vi "edit_recepie_1.vi"() -> ()   [LabVIEW 2009]
panel:
  in  "Delete":bool caption="OK2"
  in  "OK":bool caption="OK2"
  in  "Cancel":bool
  in  "path":path=path "D:/System Files/Recipe"
  out "Recipe_path":string
  in  "Recipe":i32(listbox)
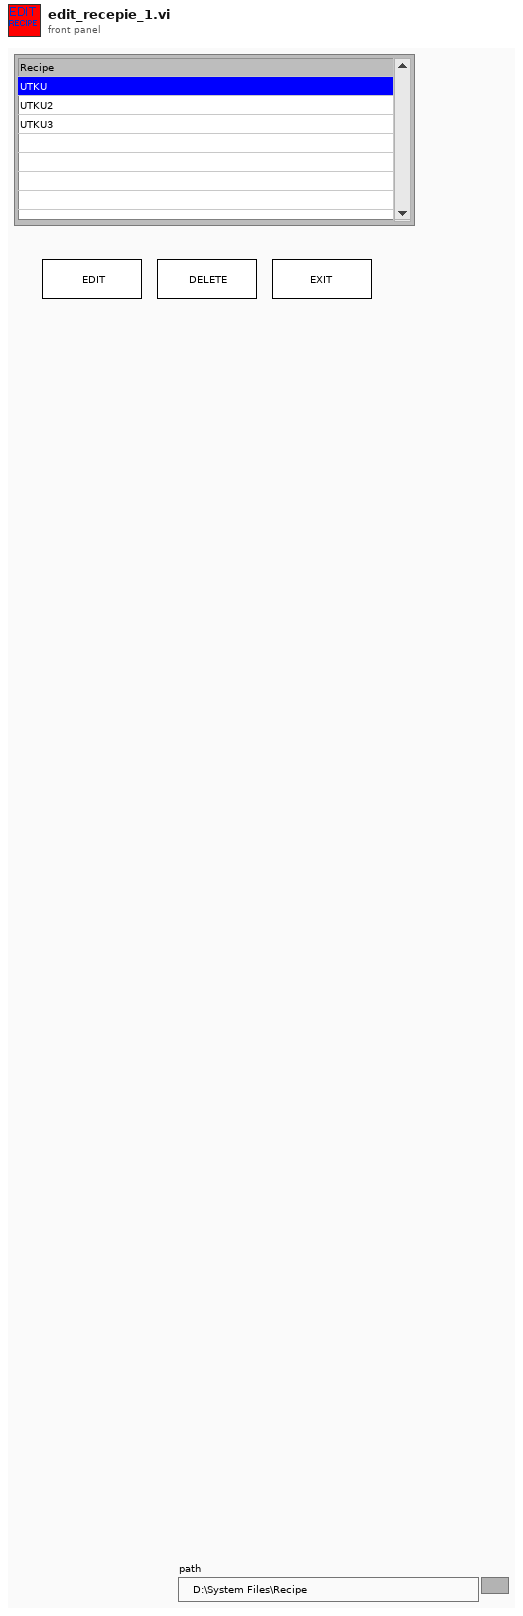
[diagram p1: front panel]
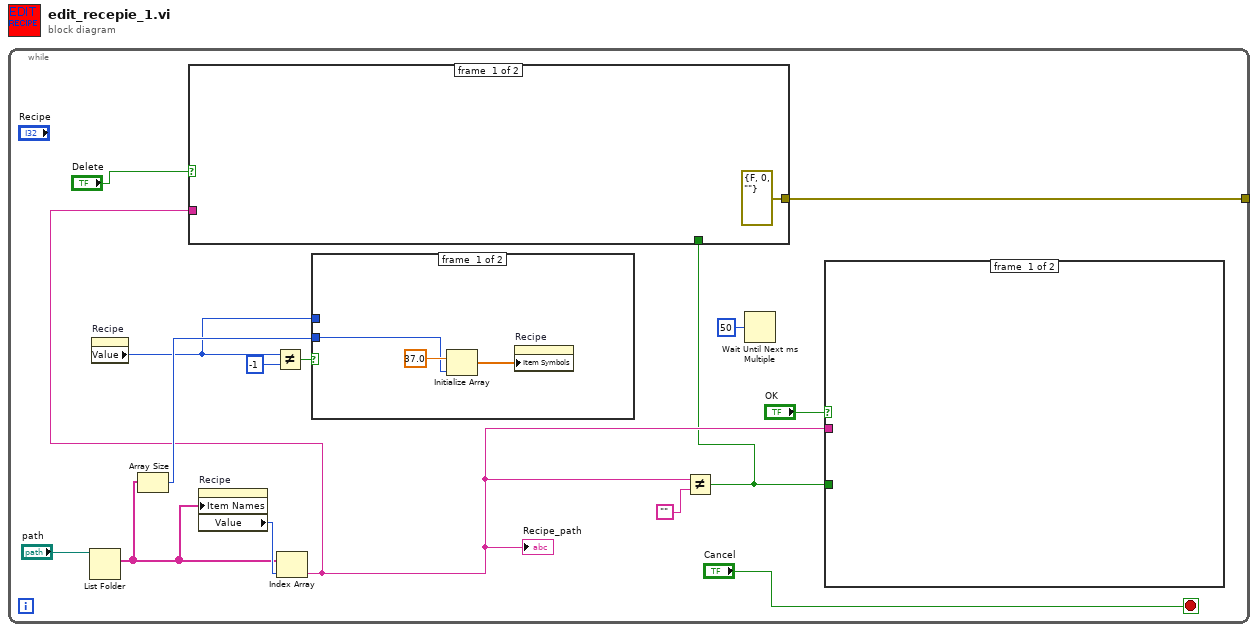
[diagram p0: block diagram]
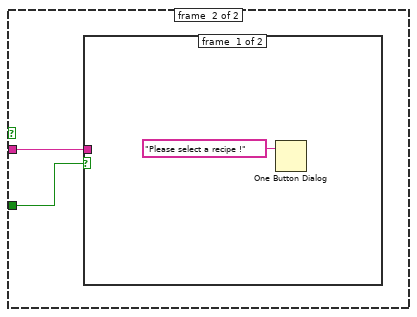
[diagram p2: hidden frame]
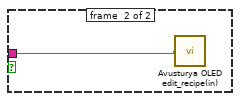
[diagram p3: hidden frame]
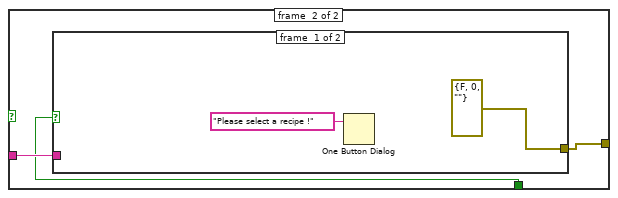
[diagram p4: hidden frame]
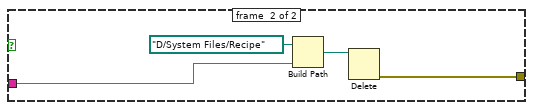
[diagram p5: hidden frame]
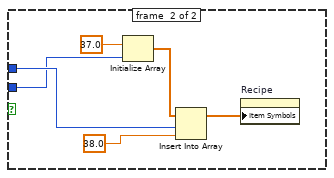
[diagram p6: hidden frame]
diagram:
  n1 = while {
    tunnel: [w1] -> _
    stop <- "Cancel" stop-if-true
    n2 = List Folder(path="path") -> (filenames=w8:string[])  [unwired: 3 in, 3 out]
    n3 = property on="Recipe" class="LstBox (strict)"() -> ("Value"=w6:i32)  [unwired: 2 in, 2 out]
    n4 = Array Size(array=w8) -> (size(s)=w7:i32)
    n5 = property on="Recipe" class="LstBox (strict)"("Item Names"=w8) -> ("Value"=w12:i32)  [unwired: 2 in, 2 out]
    n6 = Not Equal?(x=w6, y=-1) -> (x != y?=w14:bool)
    n7 = Index Array(array=w8, index=w12) -> (element=w4:string)
    "Recipe_path" <- w4
    n8 = case shown="True" w14 {
      tunnel: w6 -> [_ w35]
      tunnel: w7 -> [w31 w34]
      frame #0 {
        n9 = Initialize Array(37.0 ("element"), w31) -> (w30:dbl[])
        n10 = property on="Recipe" class="LstBox (strict)"("Item Symbols"=w30) -> ()  [unwired: 2 in, 2 out]
      }
      frame #1 {
        n11 = Initialize Array(37.0 ("element"), w34) -> (w38:dbl[])
        n12 = Insert Into Array(array=w38, index=w35, new element=38.0 ("element")) -> (w33:dbl[])
        n13 = property on="Recipe" class="LstBox (strict)"("Item Symbols"=w33) -> ()  [unwired: 2 in, 2 out]
      }
    }
    n14 = Not Equal?(x=w4, y="") -> (x != y?=w2:bool)
    n15 = case shown="False" "Delete" {
      tunnel: w4 -> [_ w23]
      tunnel: w2 -> [_ w22]
      tunnel: [errorcluster {"status"=FALSE, "code"=0, "source"=""} ("error out") w21] -> w1
      frame #0 {
      }
      frame #1 {
        n16 = case shown="False" w22 {
          tunnel: w23 -> [_ w29]
          tunnel: [errorcluster {"status"=FALSE, "code"=0, "source"=""} ("error out") w26] -> w21
          frame #0 {
            n17 = One Button Dialog(message="Please select a recipe !") -> ()  [unwired: 1 in, 1 out]
          }
          frame #1 {
            n18 = Build Path(base path=path "D:/System Files/Recipe", name or relative path=w29) -> (appended path=w28:path)
            n19 = Delete(path (use dialog)=w28) -> (error out=w26:errorcluster)  [unwired: 4 in, 2 out]
          }
        }
      }
    }
    n20 = Wait Until Next ms Multiple(millisecond multiple=u32 50) -> ()  [unwired: 1 out]
    n21 = case shown="True" "OK" {
      tunnel: w4 -> [_ w17]
      tunnel: w2 -> [_ w16]
      frame #0 {
      }
      frame #1 {
        n22 = case shown="True" w16 {
          tunnel: w17 -> [_ w19]
          frame #0 {
            n23 = One Button Dialog(message="Please select a recipe !") -> ()  [unwired: 1 in, 1 out]
          }
          frame #1 {
            n24 = call "Avusturya OLED edit_recipe(in).vi"("Path"=w19) -> ()
          }
        }
      }
    }
  }
